vi "get_all_vars.vi"(6 "timeout (ms)":i32=10000, 7 "IP address":string, 8 "error in (no error)":errorcluster, 9 "token cluster in":T1, 11 "client handle":T2) -> (0 "error out":errorcluster, 1 "token cluster":T1, 2 "variables (JSON)":string, 3 "client handle out":T2)   [LabVIEW 2018]
uses:
  <vilib>/httpClient/ClientHandle.ctl
  <vilib>/httpClient/LabVIEWHTTPClient.lvlib
panel:
  out "headers":string
  out "status code":string
  out "msg":string
  out "reponse":string
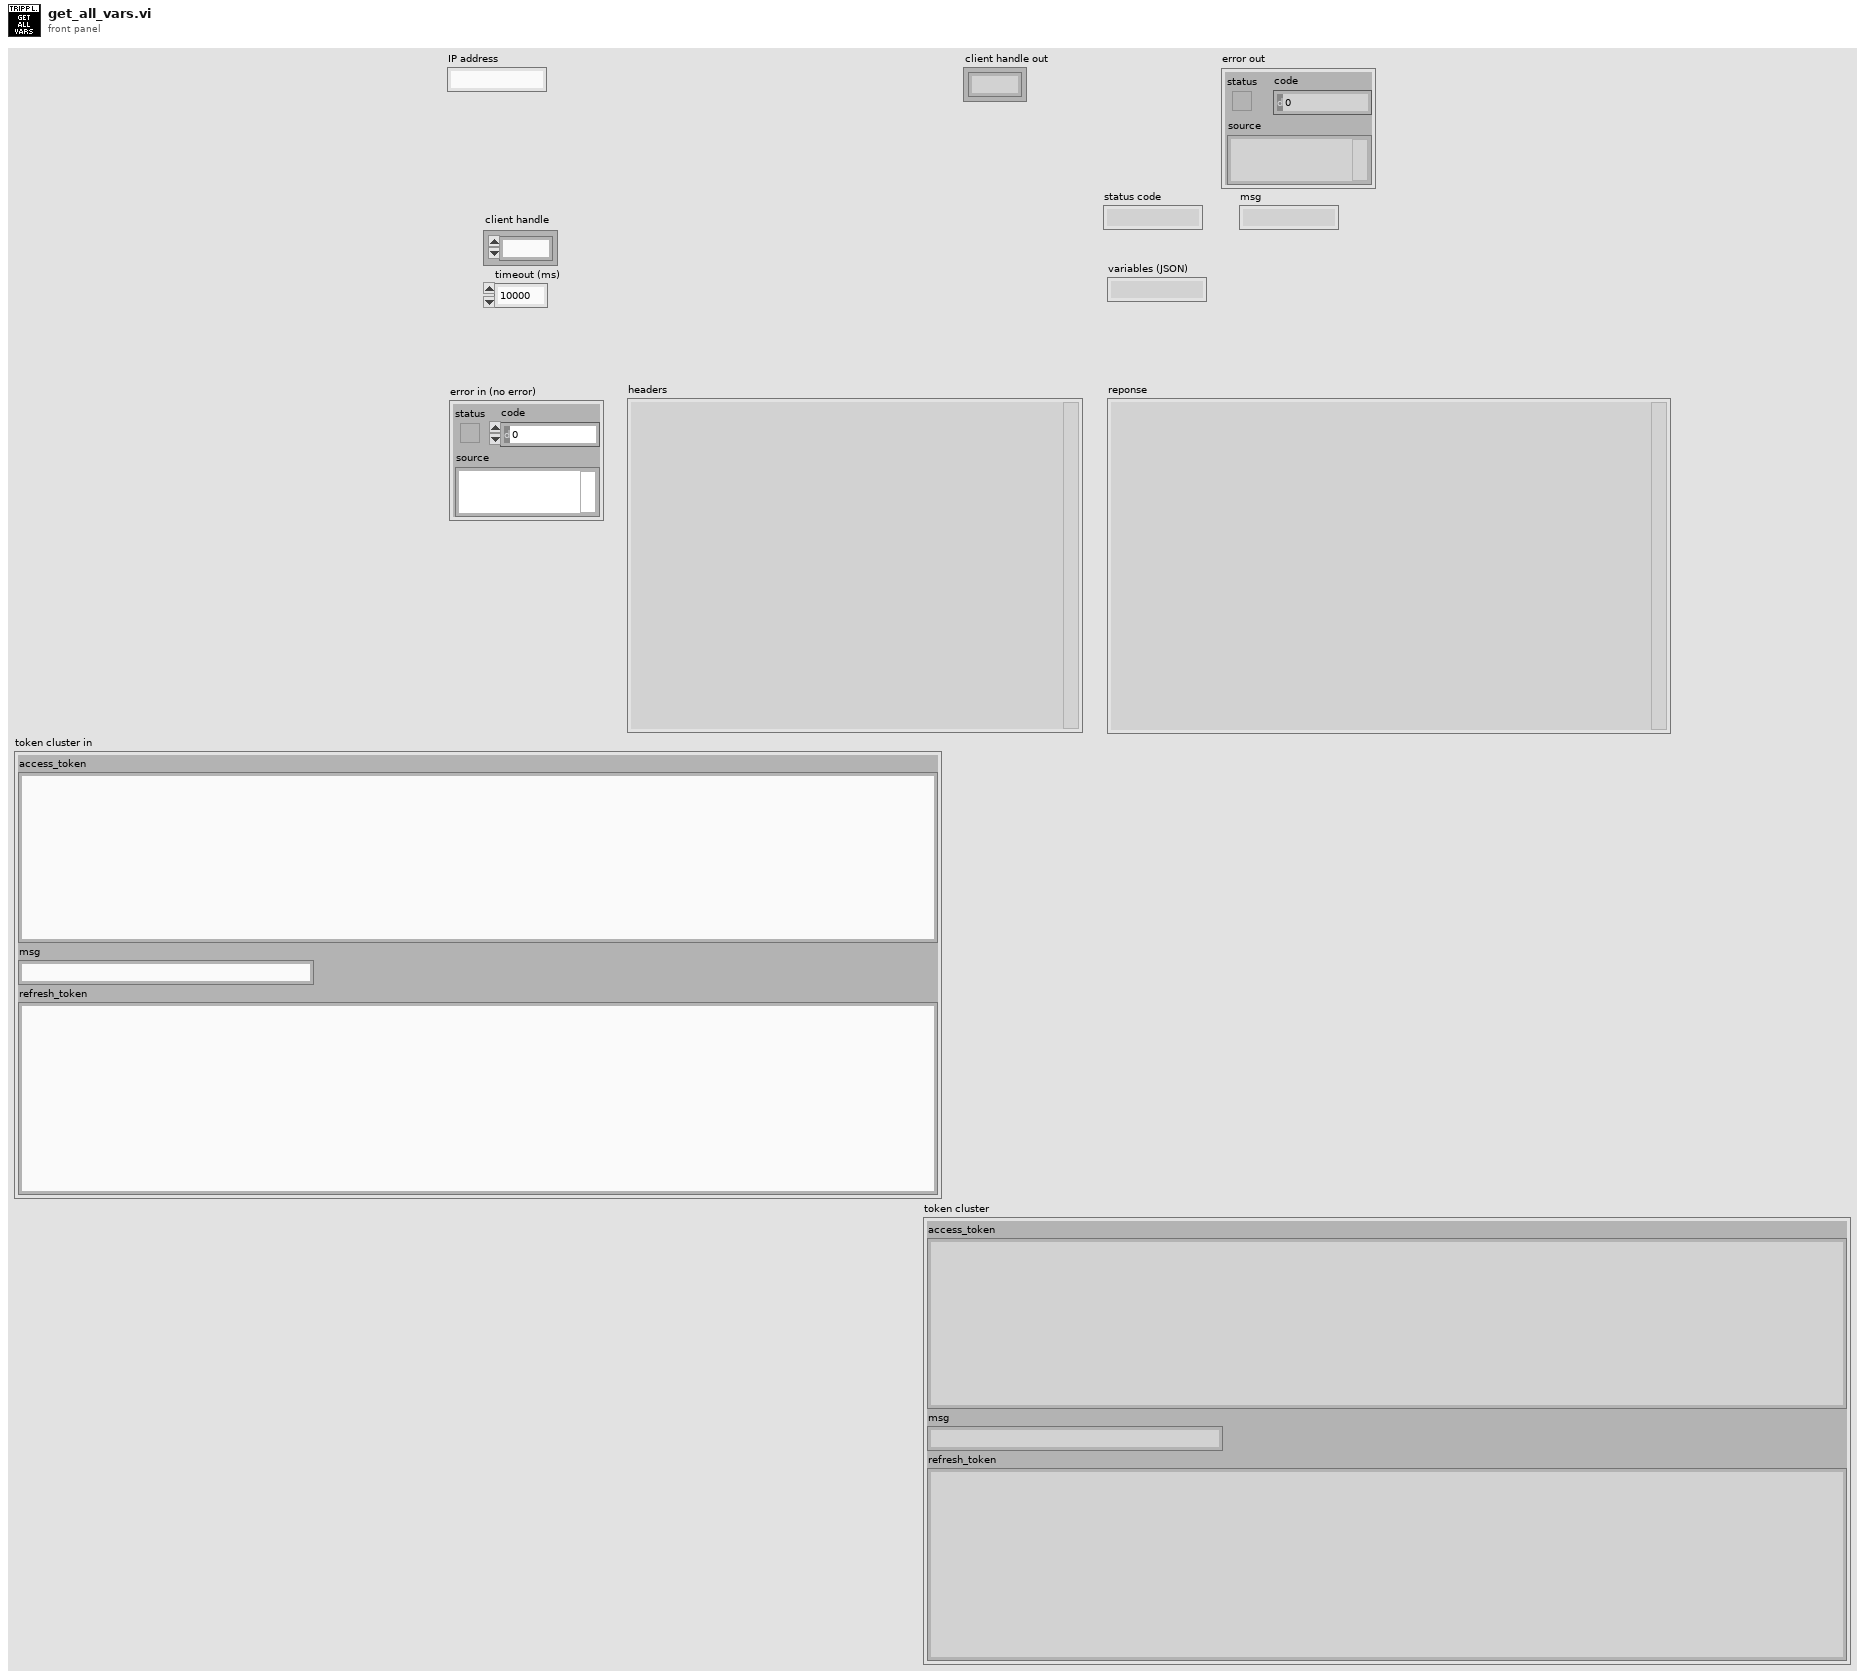
[diagram p1: front panel]
types:
  T1 = cluster{"access_token":string, "msg":string, "refresh_token":string}
  T2 = typedef "LabVIEWHTTPClient.lvlib/ClientHandle.ctl" = refnum<k1>
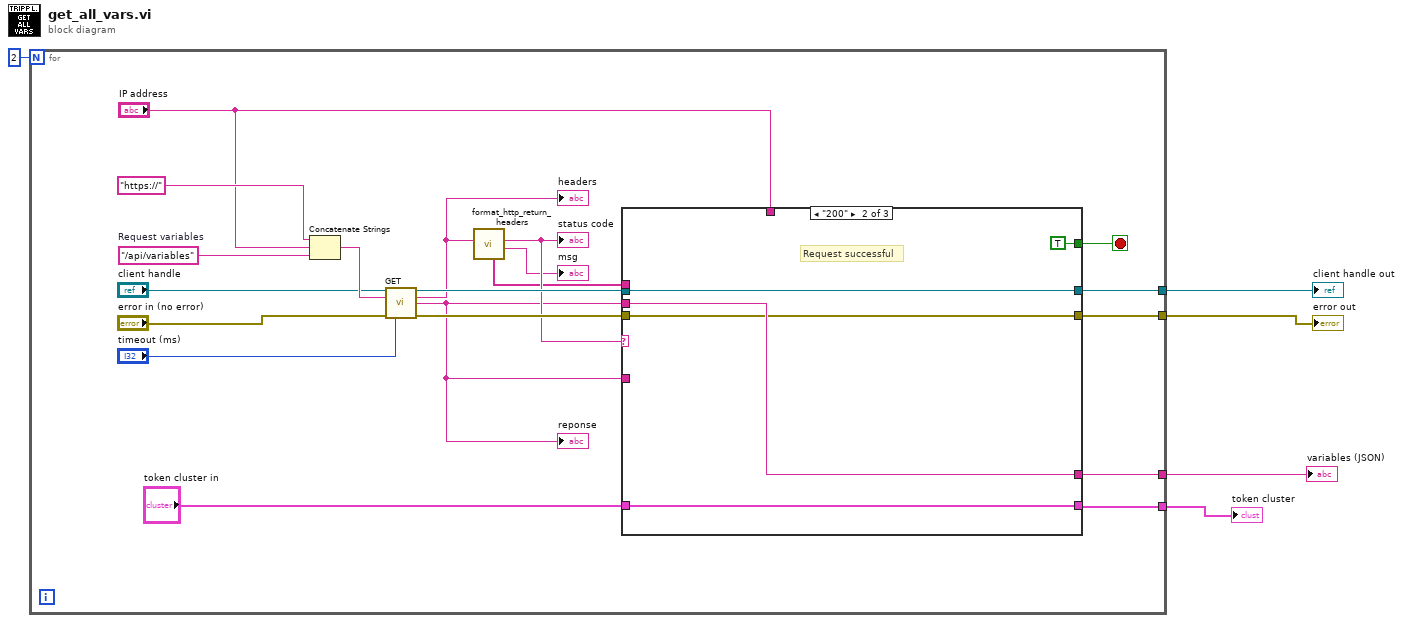
[diagram p0: block diagram]
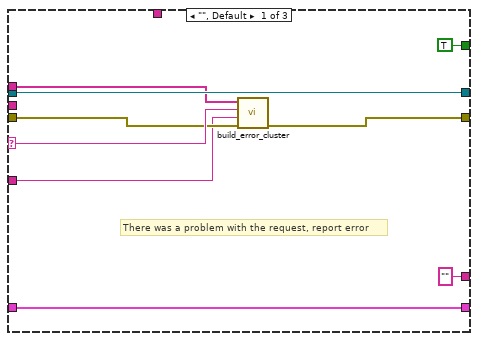
[diagram p2: hidden frame]
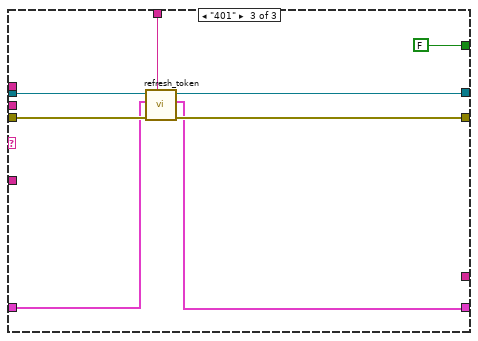
[diagram p3: hidden frame]
diagram:
  n1 = for {
    N: 2 -> [_]
    tunnel: [w20] -> w5
    tunnel: [w19] -> w4
    tunnel: [w11] -> w3
    tunnel: [w7] -> w1
    stop <- w6 stop-if-true
    w22 = "/api/variables"  # Request variables
    n2 = Concatenate Strings("https://", "IP address", w22) -> (w25:string)
    n3 = call <vilib>:"GET.vi"("client handle"="client handle", "url"=w25, "error in (no error)"="error in (no error)", "timeout (10000)"="timeout (ms)") -> ("client handle out"=w23:T2, "headers"=w18:string, "body"=w10:string, "error out"=w24:errorcluster)  [unwired: 8 in]
    "reponse" <- w10
    "headers" <- w18
    n4 = call "format_http_return_headers.vi"("headers in"=w18) -> ("msg"=→"msg":string, "status code"=w17:string, "headers array"=w15:string[])  [unwired: 8 in]
    "status code" <- w17
    n5 = case shown="\"200\"" w17 {
      selector: w17 -> [w33 _ _]
      tunnel: w24 -> [w31 w37 w47]
      tunnel: w10 -> [_ w39 _]
      tunnel: w23 -> [w34 w38 w44]
      tunnel: [w30 w37 w46] -> w20
      tunnel: [w34 w38 w45] -> w19
      tunnel: ["" ("body") w39 _] -> w11
      tunnel: w15 -> [w32 _ _]
      tunnel: w10 -> [w28 _ _]
      tunnel: "IP address" -> [_ _ w43]
      tunnel: "token cluster in" -> [w26 w35 w42]
      tunnel: [w26 w35 w41] -> w7
      tunnel: [TRUE TRUE FALSE] -> w6
      frame "", Default {
        # "There was a problem with the request, report error"
        n6 = call "build_error_cluster.vi"("error in (no error)"=w31, "error msg (JSON)"=w28, "status code"=w33, "headers array"=w32) -> ("error out"=w30:errorcluster)  [unwired: 7 in]
      }
      frame "200" {
        # "Request successful"
      }
      frame "401" {
        n7 = call "refresh_token.vi"("IP address"=w43, "error in (no error)"=w47, "token cluster in"=w42, "client handle"=w44) -> ("error out"=w46:errorcluster, "token cluster"=w41:T1, "client handle out"=w45:T2)  [unwired: 5 in]
      }
    }
  }
  "error out" <- w5
  "client handle out" <- w4
  "variables (JSON)" <- w3
  "token cluster" <- w1
